vi "testPICINPCI.vi"() -> ()   [LabVIEW 2011]
panel:
  out "Image Dst Out":T1(plugin-control)
  in  "z 3":dbl[][](graph)
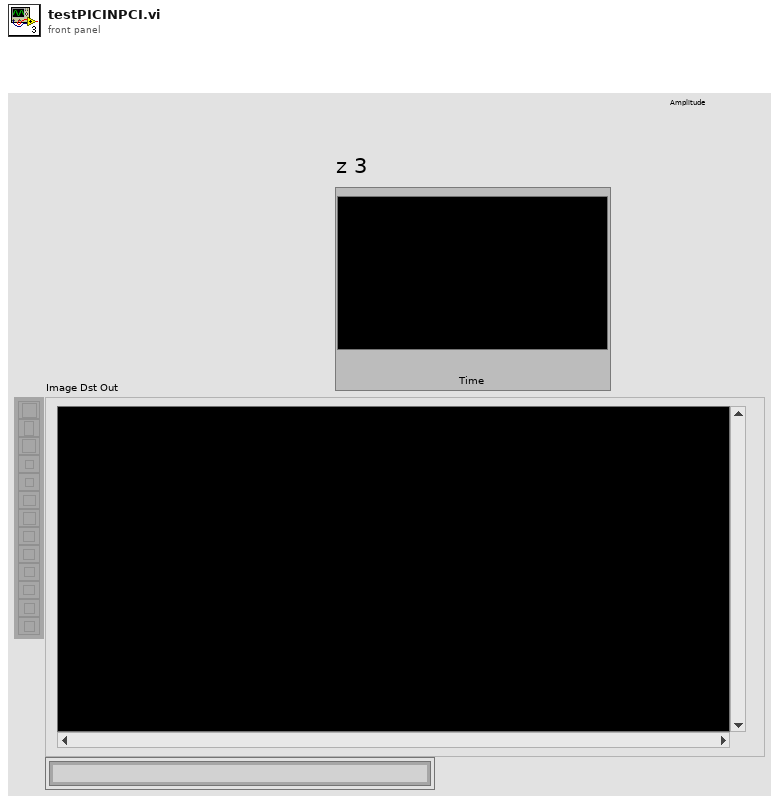
[diagram p1: front panel]
types:
  T1 = typedef "IMAQ Image.ctl" = refnum<image>
  T2 = typedef "Image Type" = u32
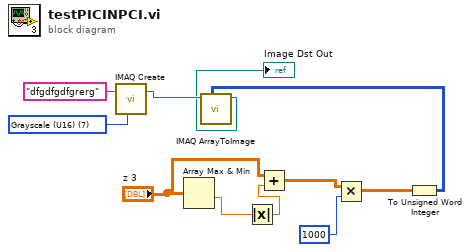
[diagram p0: block diagram]
diagram:
  w10 = T2 7 items=["Grayscale (U8)", "Grayscale (I16)", "Grayscale (SGL)", "Complex (CSG)", "RGB (U32)", "HSL (U32)", "RGB (U64)", "Grayscale (U16)"] ("Image Type")
  n1 = call "IMAQ Create"("Image Name"="dfgdfgdfgrerg", "Image Type"=w10) -> ("New Image"=w9:T1)  [unwired: 3 in, 1 out]
  n2 = Array Max & Min(array="z 3") -> (min value=w7:dbl)  [unwired: 3 out]
  n3 = Absolute Value(x=w7) -> (abs(x)=w6:dbl)
  n4 = Add(x="z 3", y=w6) -> (x+y=w4:dbl[][])
  n5 = Multiply(x=w4, y=1000) -> (x*y=w2:dbl[][])
  n6 = To Unsigned Word Integer(number=w2) -> (unsigned 16bit integer=w1:u16[][])
  n7 = call "IMAQ ArrayToImage"("Image Pixels (U16)"=w1, "Image"=w9) -> ("Image Out"=→"Image Dst Out":T1)  [unwired: 8 in, 1 out]
